vi "FGVFileServer.vi"(7 "Enum":T1, 8 "error in":errorcluster, 10 "New VI":string, 11 "ViIn":string[](array[string])) -> (0 "error out":errorcluster, 3 "VIOut":string[](array[string]))   [LabVIEW 2016]
uses:
  controls/EnumFGVHDT.ctl
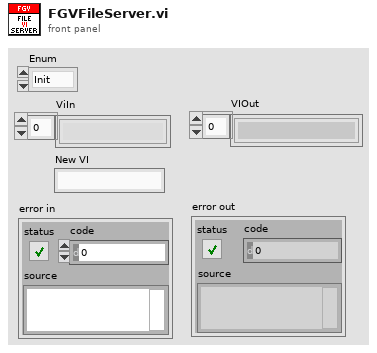
[diagram p1: front panel]
types:
  T1 = typedef "EnumFGVHDT.ctl" = enum16{"Init", "Read", "Write", "Push", "Pop"}
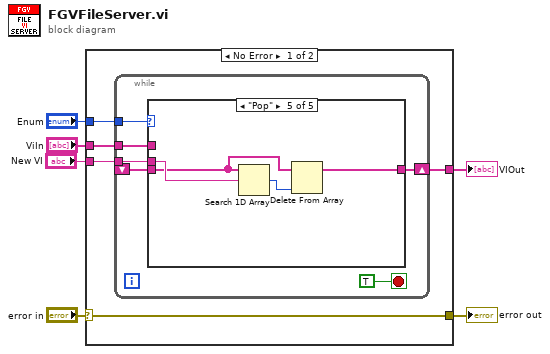
[diagram p0: block diagram]
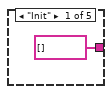
[diagram p2: hidden frame]
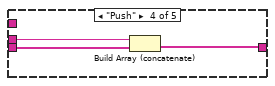
[diagram p5: hidden frame]
diagram:
  n1 = case shown="No Error" "error in" {
    selector: "error in" -> [w10 w29]
    tunnel: "Enum" -> [w11 _]
    tunnel: [w10 w29] -> w6
    tunnel: "ViIn" -> [w8 w28]
    tunnel: [w9 w28] -> w3
    tunnel: "New VI" -> [w7 _]
    frame No Error {
      n2 = while {
        tunnel: w11 -> [w16]
        tunnel: w8 -> [w14]
        shift-right: [w15] -> w9
        shift-left: _ -> [w13]
        tunnel: w7 -> [w12]
        stop <- TRUE stop-if-true
        n3 = case shown="\"Pop\"" w16 {
          tunnel: [string[] [] ("OwnerViIn") w19 w20 w23 w27] -> w15
          tunnel: w14 -> [_ _ w20 _ _]
          tunnel: w13 -> [_ w19 _ w22 w24]
          tunnel: w12 -> [_ _ _ w21 w26]
          frame "Init" {
          }
          frame "Read", Default {
          }
          frame "Write" {
          }
          frame "Push" {
            n4 = Build Array (concatenate)(w21, w22) -> (w23:string[])
          }
          frame "Pop" {
            n5 = Search 1D Array(1D array=w24, element=w26) -> (index of element=w25:i32)  [unwired: 1 in]
            n6 = Delete From Array(array=w24, index=w25) -> (array with subset deleted=w27:string[])  [unwired: 1 in, 1 out]
          }
        }
      }
    }
    frame Error {
    }
  }
  "error out" <- w6
  "VIOut" <- w3
